vi "communicatie met arduino.vi"() -> ()   [LabVIEW 2023]
uses:
  <vilib>/Instr/_visa.llb/VISA Configure Serial Port (Instr).vi
panel:
  in  "stop":bool
  out "Hoek waterstraal":dbl
  out "om te testen wat de output van de arduino is":string
  in  "Manueel?":bool
  out "Watersnelheid (L/min)":dbl
  out "Totale hoeveelheid uitgespoten water (mL)":dbl
  out "standard output":string
  out "standard error":string
  out "return code na runnen python programma":i32
  in  "VISA resource name":refnum<visa-resource-name>
  # "ALLES VOOR AUTOMATISCH RUNNEN VAN PYTHON PROGRAMMA"
  # "ALLES VOOR AUTOMATISCHE WERKING"
  # "ALLES VOOR MANUELE BESTURING"
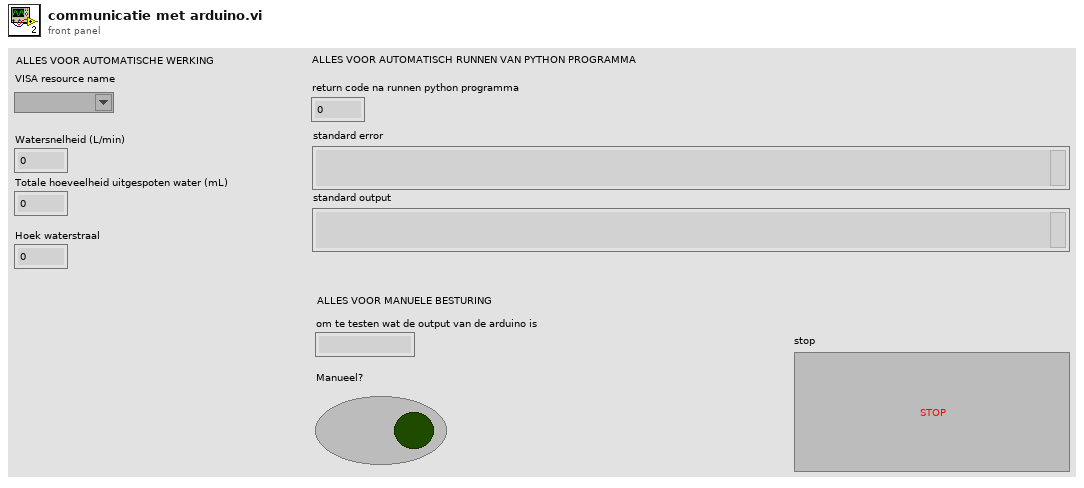
[diagram p1: front panel]
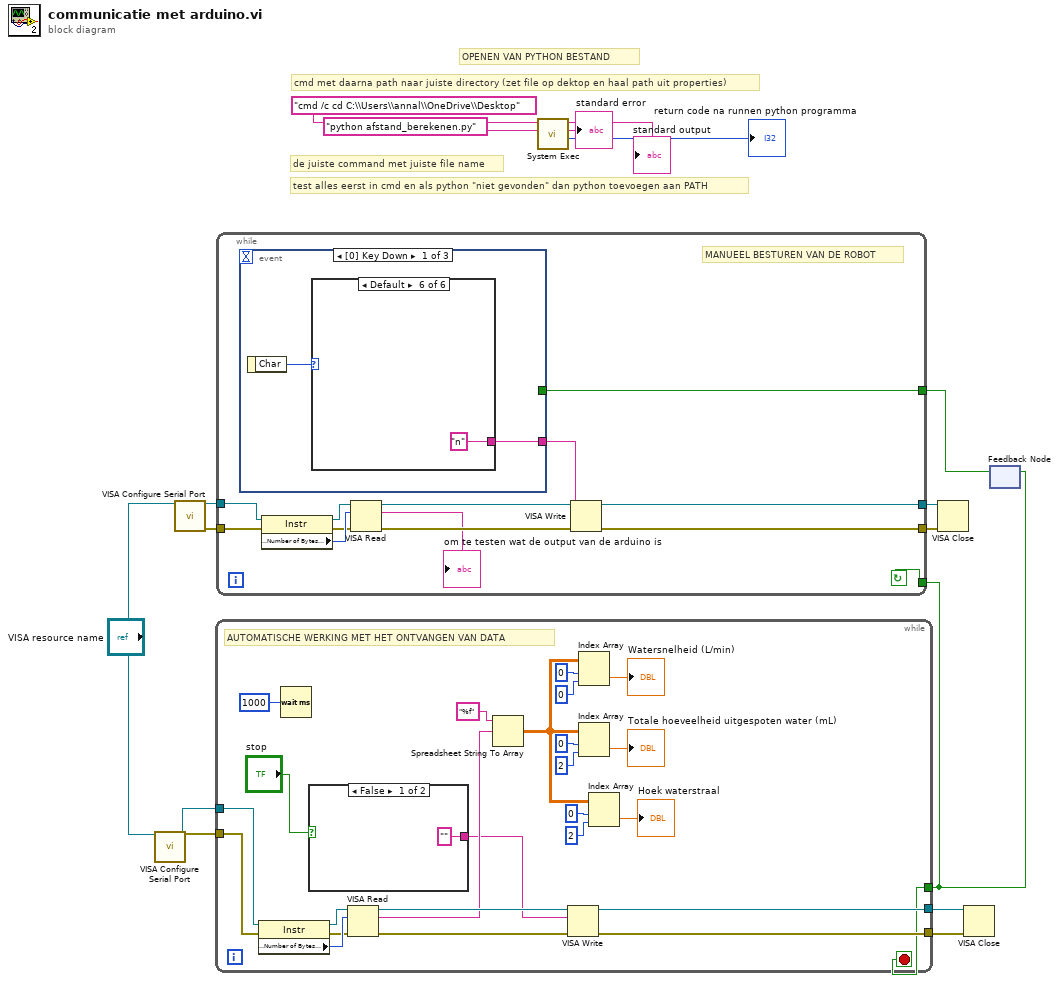
[diagram p0: block diagram]
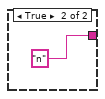
[diagram p2: hidden frame]
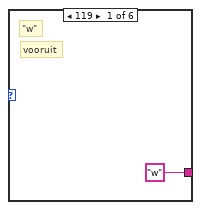
[diagram p3: hidden frame]
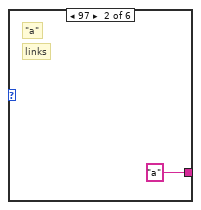
[diagram p4: hidden frame]
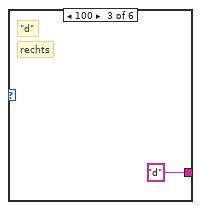
[diagram p5: hidden frame]
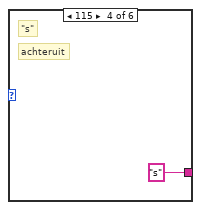
[diagram p6: hidden frame]
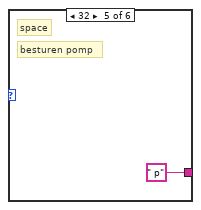
[diagram p7: hidden frame]
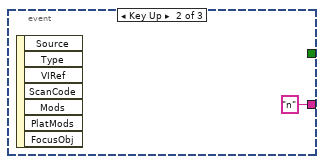
[diagram p8: hidden frame]
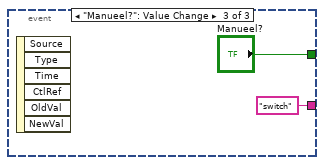
[diagram p9: hidden frame]
diagram:
  # "test alles eerst in cmd en als python \"niet gevonden\" dan python toevoegen aan PATH"
  # "OPENEN VAN PYTHON BESTAND"
  # "de juiste command met juiste file name"
  # "cmd met daarna path naar juiste directory (zet file op dektop en haal path uit properties)"
  n1 = call-poly "VISA Configure Serial Port"("VISA resource name"="VISA resource name") -> ("VISA resource name out"=w7:refnum<visa-resource-name>, "error out"=w6:errorcluster)  [unwired: 13 in]
  n2 = call-poly "VISA Configure Serial Port"("VISA resource name"="VISA resource name") -> ("VISA resource name out"=w16:refnum<visa-resource-name>, "error out"=w15:errorcluster)  [unwired: 13 in]
  n3 = call <vilib>:"System Exec.vi"("standard input"="python afstand_berekenen.py", "command line"="cmd /c cd C:\\Users\\annal\\OneDrive\\Desktop") -> ("return code"=→"return code na runnen python programma":i32, "standard error"=→"standard error":string, "standard output"=→"standard output":string)  [unwired: 6 in, 1 out]
  n4 = feedback #1() -> (w1:bool)  [unwired: 1 in]
  n5 = while {
    tunnel: w7 -> [w39]
    tunnel: w6 -> [w38]
    tunnel: [w41] -> w5
    tunnel: [w40] -> w4
    tunnel: w1 -> [w23]
    stop <- w23 stop-if-true
    # "AUTOMATISCHE WERKING MET HET ONTVANGEN VAN DATA"
    n6 = property class="Instr"(reference=w39, error in=w38) -> (reference out=w35:refnum<visa-resource-name>, error out=w36:errorcluster, "Serial Settings:Number of Bytes at Serial Port"=w37:u32)
    n7 = Wait (ms)(milliseconds to wait=u32 1000) -> ()  [unwired: 1 out]
    n8 = case shown="False" "stop" {
      tunnel: ["" "n"] -> w17
      frame False {
      }
      frame True {
      }
    }
    n9 = VISA Read(VISA resource name=w35, byte count=w37, error in (no error)=w36) -> (VISA resource name out=w34:refnum<visa-resource-name>, read buffer=w24:string, error out=w33:errorcluster)  [unwired: 1 out]
    n10 = Spreadsheet String To Array(format string="%f", spreadsheet string=w24) -> (array=w19:dbl[][])  [unwired: 2 in]
    n11 = VISA Write(VISA resource name=w34, write buffer=w17, error in (no error)=w33) -> (VISA resource name out=w40:refnum<visa-resource-name>, error out=w41:errorcluster)  [unwired: 1 out]
    n12 = Index Array(array=w19, index (row)=0, index (col)=0 ("disabled index (col)")) -> (element=→"Watersnelheid (L/min)":dbl)
    n13 = Index Array(array=w19, index (row)=0, index (col)=2 ("disabled index (col)")) -> (element=→"Totale hoeveelheid uitgespoten water (mL)":dbl)
    n14 = Index Array(array=w19, index (row)=0, index (col)=2 ("disabled index (col)")) -> (element=→"Hoek waterstraal":dbl)
  }
  n15 = while {
    tunnel: w16 -> [w54]
    tunnel: w15 -> [w53]
    tunnel: [w56] -> w14
    tunnel: [w55] -> w13
    tunnel: w1 -> [w46]
    tunnel: [w44] -> w2
    stop <- w46 continue-if-true
    # "MANUEEL BESTUREN VAN DE ROBOT"
    n16 = event shown="[0] Key Down" {
      selector: _ -> [_ _ _]
      dyn-events: _ -> [_ _ _]
      timeout: _ -> [_ _ _]
      tunnel: [w58 "n" ("write buffer") "switch" ("write buffer")] -> w47
      tunnel: [_ _ "Manueel?"] -> w44
      event Key Down {
        n17 = event-data() -> ("Char"=w57:i16)  [unwired: 1 in]
        n18 = case shown="Default" w57 {
          tunnel: ["w" ("write buffer") "a" ("write buffer") "d" ("write buffer") "s" ("write buffer") " p" ("write buffer") "n" ("write buffer")] -> w58
          frame 119 {
            # "vooruit"
            # "\"w\""
          }
          frame 97 {
            # "links"
            # "\"a\""
          }
          frame 100 {
            # "rechts"
            # "\"d\""
          }
          frame 115 {
            # "achteruit"
            # "\"s\""
          }
          frame 32 {
            # "besturen pomp"
            # "space"
          }
          frame Default {
          }
        }
      }
      event Key Up {
        n19 = event-data() -> ()  [unwired: 1 in, 7 out]
      }
      event "Manueel?": Value Change {
        n20 = event-data() -> ()  [unwired: 1 in, 6 out]
      }
    }
    n21 = property class="Instr"(reference=w54, error in=w53) -> (reference out=w50:refnum<visa-resource-name>, error out=w51:errorcluster, "Serial Settings:Number of Bytes at Serial Port"=w52:u32)
    n22 = VISA Read(VISA resource name=w50, byte count=w52, error in (no error)=w51) -> (VISA resource name out=w49:refnum<visa-resource-name>, read buffer=→"om te testen wat de output van de arduino is":string, error out=w48:errorcluster)  [unwired: 1 out]
    n23 = VISA Write(VISA resource name=w49, write buffer=w47, error in (no error)=w48) -> (VISA resource name out=w55:refnum<visa-resource-name>, error out=w56:errorcluster)  [unwired: 1 out]
  }
  n24 = VISA Close(VISA resource name=w13, error in (no error)=w14) -> ()  [unwired: 1 out]
  n25 = VISA Close(VISA resource name=w4, error in (no error)=w5) -> ()  [unwired: 1 out]
  n26 = feedback-in #1(w2) -> ()
